vi "JLINKARM Write U16.vi"(8 "error in (no error)":errorcluster caption="错误输入（无错误）", 10 "data":u16, 11 "memaddr":u32) -> (0 "error out":errorcluster caption="错误输出", 3 "function return":i32)   [LabVIEW 2016, in "JLinkARM.lvlib"]
doc: "int JLINKARM_WriteU16(unsigned long memaddr,unsigned short int data);"
uses:
  <userlib>/LV-JLinkARM/JLinkARM.lvlib
  <userlib>/LV-JLinkARM/JLinkARM.dll
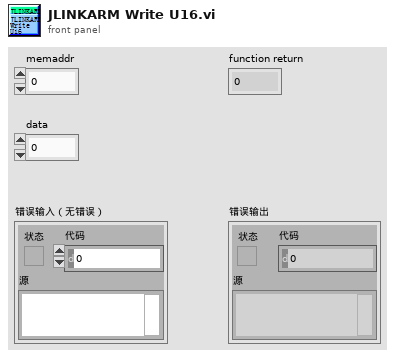
[diagram p1: front panel]
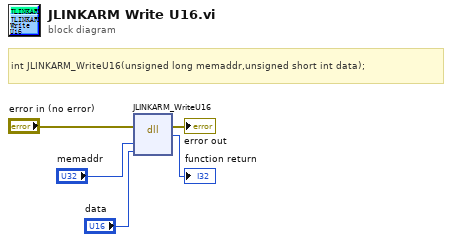
[diagram p0: block diagram]
diagram:
  # "int JLINKARM_WriteU16(unsigned long memaddr,unsigned short int data);"
  n1 = dll-call lib="C:/Program Files (x86)/National Instruments/LabVIEW 2016/user.lib/LV-JLinkARM/JLinkARM.*" fn="JLINKARM_WriteU16"(error in="error in (no error)", "memaddr"="memaddr", "data"="data") -> (error out=→"error out":errorcluster, →"function return":i32)  [unwired: 4 in, 1 out]
